vi "Init Data Object.vi"(11 "PAS Cell Data in":refnum<class "PAS Cell Data.lvclass">) -> (3 "PAS Cell Data out":refnum<class "PAS Cell Data.lvclass">)   [LabVIEW 2014, in "PAS Library.lvlib" / "PAS Cell Data.lvclass"]
uses:
  PAS Cell Data.lvclass
  Data/Data.lvclass
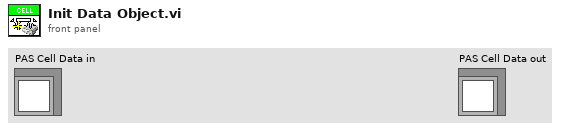
[diagram p1: front panel]
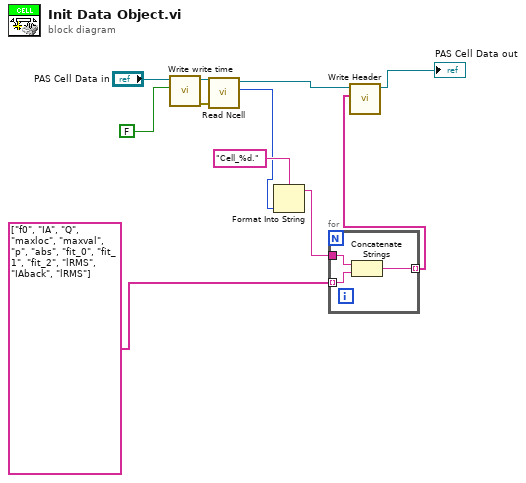
[diagram p0: block diagram]
diagram:
  n1 = call "Write write time.vi"("write time"=FALSE, "Data in"="PAS Cell Data in") -> ("error out"=w8:errorcluster, "Data out"=w9:refnum<class "PAS Cell Data.lvclass">)  [unwired: 8 in]
  n2 = call "Read Ncell.vi"("error in (no error)"=w8, "PAS Cell Data in"=w9) -> ("Ncell"=w6:u8, "PAS Cell Data out"=w3:refnum<class "PAS Cell Data.lvclass">)  [unwired: 7 in, 1 out]
  n3 = Format Into String(format string="Cell_%d.", w6) -> (resulting string=w5:string)  [unwired: 2 in, 1 out]
  n4 = for {
    tunnel: w5 -> [w14]
    tunnel: string[] ["f0", "IA", "Q", "maxloc", "maxval", "p", "abs", "fit_0", "fit_1", "fit_2", "lRMS", "IAback", "lRMS"] ("Header") -> [w13] mode=indexing
    tunnel: [w12] -> w2 mode=indexing
    n5 = Concatenate Strings(w14, w13) -> (w12:string)
  }
  n6 = call "Write Header.vi"("Header"=w2, "Data in"=w3) -> ("Data out"=→"PAS Cell Data out":refnum<class "PAS Cell Data.lvclass">)  [unwired: 8 in, 1 out]
